vi "Begin.vi"   [LabVIEW 2012]
doc: "Called before other user functions, this VI is expected to open initial I/O refnums, load in file data, and do all program initialization. Notice that the <B>error out</B> terminal is simply used for data flow. Wiring it to other structures or subVIs ensures that this VI runs first."
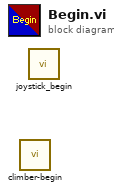
[diagram p0: block diagram]
diagram:
  n1 = call "climber-begin.vi"() -> ()  [unwired: 12 in]
  n2 = call "joystick_begin.vi"() -> ()  [unwired: 12 in]
